vi "RunExeutiveFile.vi"() -> ()   [LabVIEW 2010]
uses:
  <vilib>/Utility/file.llb/Read From Spreadsheet File (string).vi
panel:
  in  "Delimiter\n\"\\t\" for tab\n\"\",\" for comma":string="\t"
  in  "COM Port":refnum<visa-resource-name>
  in  "Exec File":path
  out "Array":string[][](array[string])
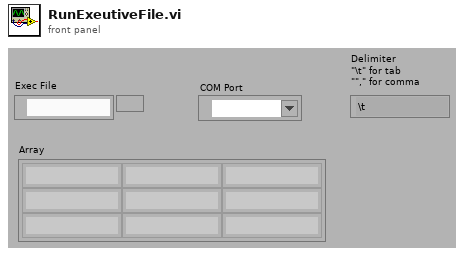
[diagram p1: front panel]
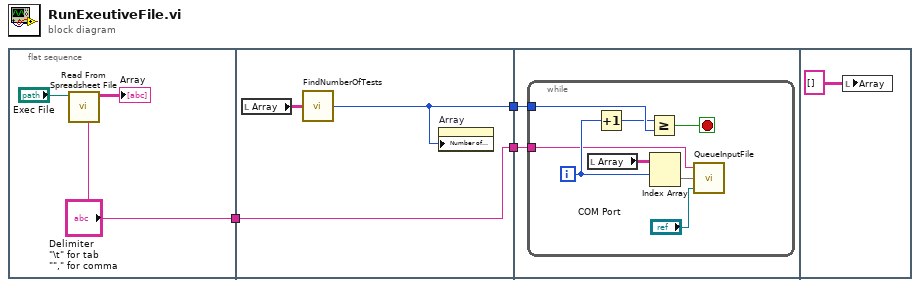
[diagram p0: block diagram]
diagram:
  n1 = flat-sequence {
    tunnel: ["Delimiter\n\"\\t\" for tab\n\"\",\" for comma"] -> w1
    tunnel: [w8] -> w3
    tunnel: [w7] -> w2
    tunnel: w1 -> [w7]
    tunnel: w3 -> [w11]
    tunnel: w2 -> [w10]
    frame #0 {
      n2 = call-poly <vilib>:"Read From Spreadsheet File.vi"("delimiter (\\t)"="Delimiter\n\"\\t\" for tab\n\"\",\" for comma", "file path (dialog if empty)"="Exec File") -> ("all rows"=→"Array":string[][])  [unwired: 5 in, 4 out]
    }
    frame #1 {
      n3 = local read "Array"() -> (w9:string[][])
      n4 = call "FindNumberOfTests.vi"("Array"=w9) -> ("Numeric"=w8:i32)
      n5 = property on="Array" class="Arr (strict)"("Number of Rows"=w8) -> ()  [unwired: 2 in, 2 out]
    }
    frame #2 {
      n6 = while {
        tunnel: w11 -> [w18]
        tunnel: w10 -> [w12]
        i -> [w13]
        stop <- w19 stop-if-true
        n7 = local read "Array"() -> (w15:string[][])
        n8 = Increment(x=w13) -> (x+1=w17:i32)
        n9 = Greater Or Equal?(x=w17, y=w18) -> (x >= y?=w19:bool)
        n10 = Index Array(array=w15, index (row)=w13) -> (element=w14:string[])  [unwired: 1 in]
        n11 = call "QueueInputFile.vi"("VISA resource name"="COM Port", "Array"=w14, "Delimiter Character"=w12) -> ()  [unwired: 1 in]
      }
    }
    frame #3 {
      n12 = local write "Array"(string[][] []) -> ()
    }
  }
